vi "String to Diag Matrix.vi"(1 "Martix Dimension":i32, 2 "String Input":string) -> (0 "Matrix Out":T1)   [LabVIEW 2011]
uses:
  <vilib>/Analysis/Matrix/Datatypes/RealMatrix.ctl
  <vilib>/Analysis/Matrix/NI_Matrix.lvlib
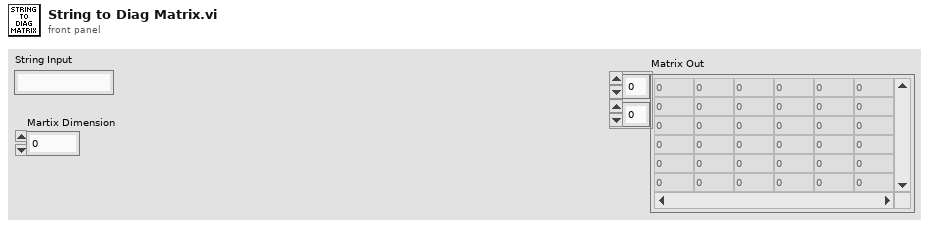
[diagram p1: front panel]
types:
  T1 = typedef "NI_Matrix.lvlib/RealMatrix.ctl" = dbl[][]
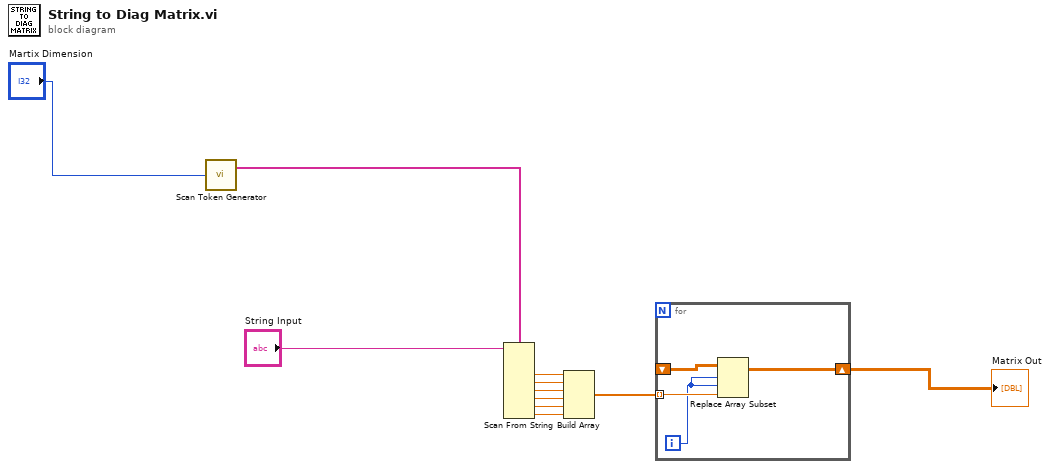
[diagram p0: block diagram]
diagram:
  n1 = call "Scan Token Generator.vi"("Martix Dimension"="Martix Dimension") -> ("Array"=w1:string[])
  n2 = Scan From String(format string=w1, input string="String Input") -> (output 1=w10:dbl, output 2=w9:dbl, output 3=w8:dbl, output 4=w7:dbl, output 5=w6:dbl, output 6=w5:dbl)  [unwired: 8 in, 3 out]
  n3 = Build Array(w10, w9, w8, w7, w6, w5) -> (w4:dbl[])
  n4 = for {
    tunnel: w4 -> [w13] mode=indexing
    shift-right: [w14] -> w3
    shift-left: _ -> [w15]
    i -> [w12]
    n5 = Replace Array Subset(array=w15, new element=w13, index (row)=w12, index (col)=w12) -> (w14:T1)
  }
  "Matrix Out" <- w3
